vi "PXI-Get Excluded Slots.vi"(7 "key":string="Excluded slots", 11 "error in (no error)":errorcluster) -> (8 "excluded slots":i32[](array[numeric]), 15 "error out":errorcluster)   [LabVIEW 2020]
uses:
  <vilib>/Utility/config.llb/Read Key (String).vi
  <vilib>/Utility/config.llb/NI_LVConfig.lvlib
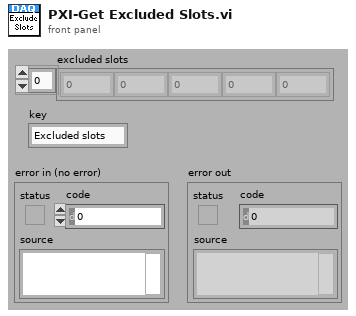
[diagram p1: front panel]
types:
  T1 = typedef "NI_LVConfig.lvlib/Config Data RefNum.ctl" = refnum<k1>
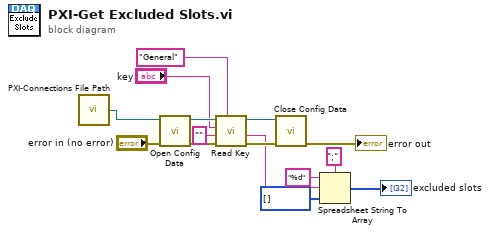
[diagram p0: block diagram]
diagram:
  n1 = call "PXI-Connections File Path.vi"() -> ("Path"=w1:path)  [unwired: 1 in]
  n2 = call <vilib>:"Open Config Data.vi"("error in (no error)"="error in (no error)", "configuration file path"=w1) -> ("error out"=w14:errorcluster, "refnum"=w13:T1)  [unwired: 7 in, 1 out]
  n3 = call-poly <vilib>:"Read Key.vi"("section"="General", "error in (no error)"=w14, "default value"="", "key"="key", "refnum"=w13) -> ("error out"=w10:errorcluster, "value"=w7:string, "refnum out"=w9:T1)  [unwired: 3 in, 1 out]
  n4 = call <vilib>:"Close Config Data.vi"("error in (no error)"=w10, "refnum"=w9) -> ("error out"=→"error out":errorcluster)  [unwired: 8 in, 1 out]
  n5 = Spreadsheet String To Array(delimiter (Tab)=";", format string="%d", spreadsheet string=w7, array type (2D Dbl)=i32[] []) -> (array=→"excluded slots":i32[])
